vi "Add file.vi"(8 "error in (no error)":errorcluster, 9 "Insert in front":bool, 10 "File Path Control":path, 11 "MagLabGraph in":refnum<class "MagLabGraph.lvclass">) -> (0 "error out":errorcluster, 3 "MagLabGraph out":refnum<class "MagLabGraph.lvclass">)   [LabVIEW 2015, in "MagLabGraph.lvclass"]
uses:
  MagLabGraph.lvclass
  <vilib>/ActorFramework/Actor/Actor.lvclass/Actor.ctl
  <vilib>/ActorFramework/Message Enqueuer/Message Enqueuer.lvclass/Message Enqueuer.ctl
  MagLabGraph Messages/Add file Msg/Add file Msg.lvclass/Add file Msg.ctl
  MagLabGraph.lvclass/MagLabGraph.ctl
  <vilib>/ActorFramework/Message Enqueuer/Init from Existing Queue.vi
  <vilib>/ActorFramework/Time-Delayed Send Message/Time-Delayed Send Message.vi
  <vilib>/ActorFramework/Message Enqueuer/Message Enqueuer.lvclass
  MagLabGraph Messages/Add file Msg/Add file Msg.lvclass
  <vilib>/ActorFramework/Actor/Actor.lvclass
  Mag Lab Error Handler/Mag Lab Error Handler.lvclass
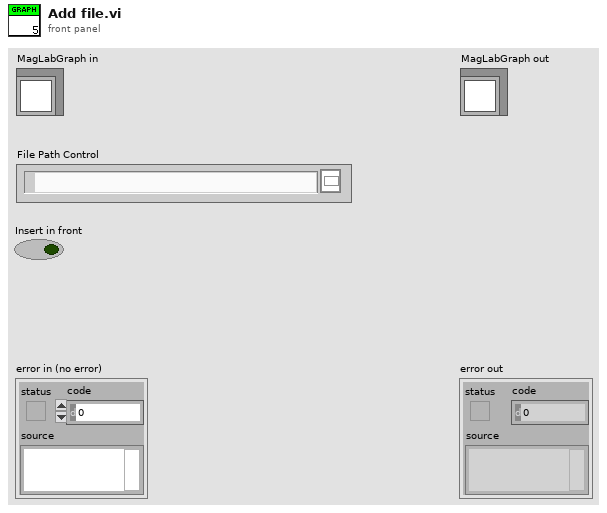
[diagram p1: front panel]
types:
  T1 = typedef "File_Group_Chan_Abbr.ctl" = cluster{"File Path Control":path, "Group":string, "Channel":string, "Abbreviated":string}
  T2 = cluster{"File Path Control":path, "Group":string, "Channel":string, "Abbreviated":string}[]
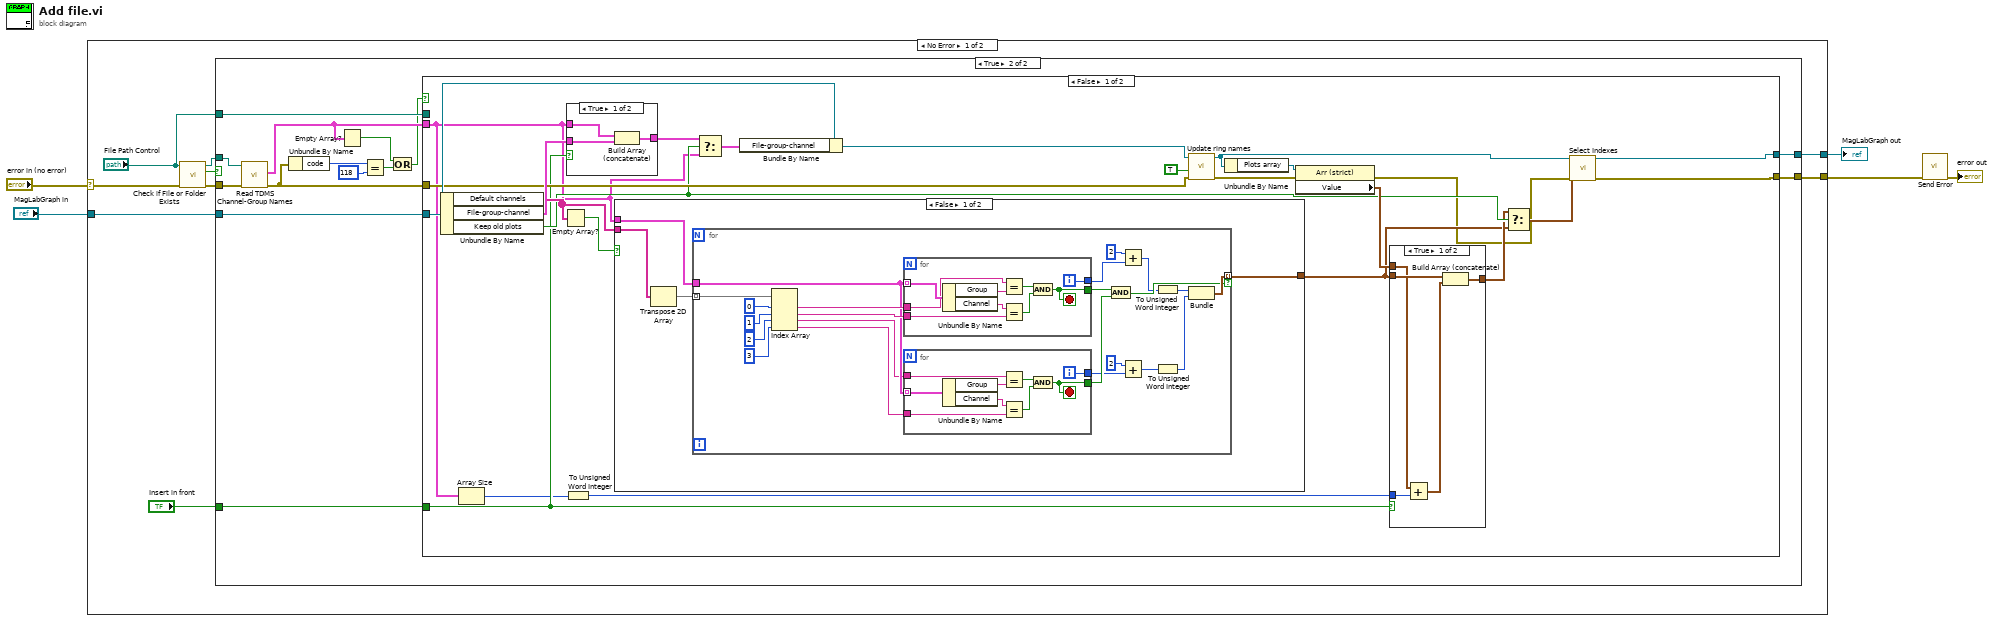
[diagram p0: block diagram]
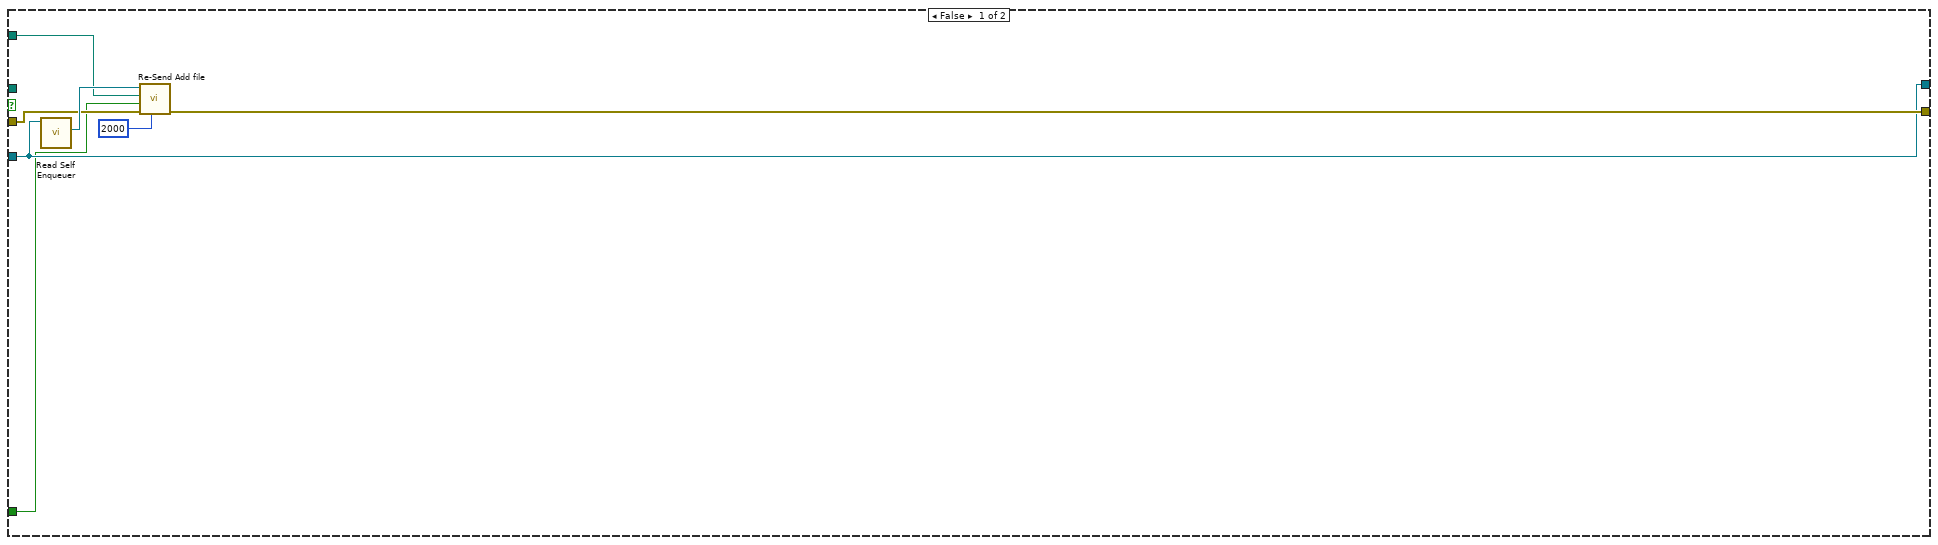
[diagram p2: hidden frame]
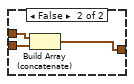
[diagram p3: hidden frame]
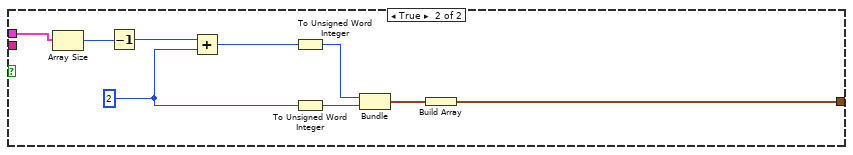
[diagram p4: hidden frame]
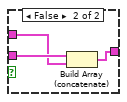
[diagram p5: hidden frame]
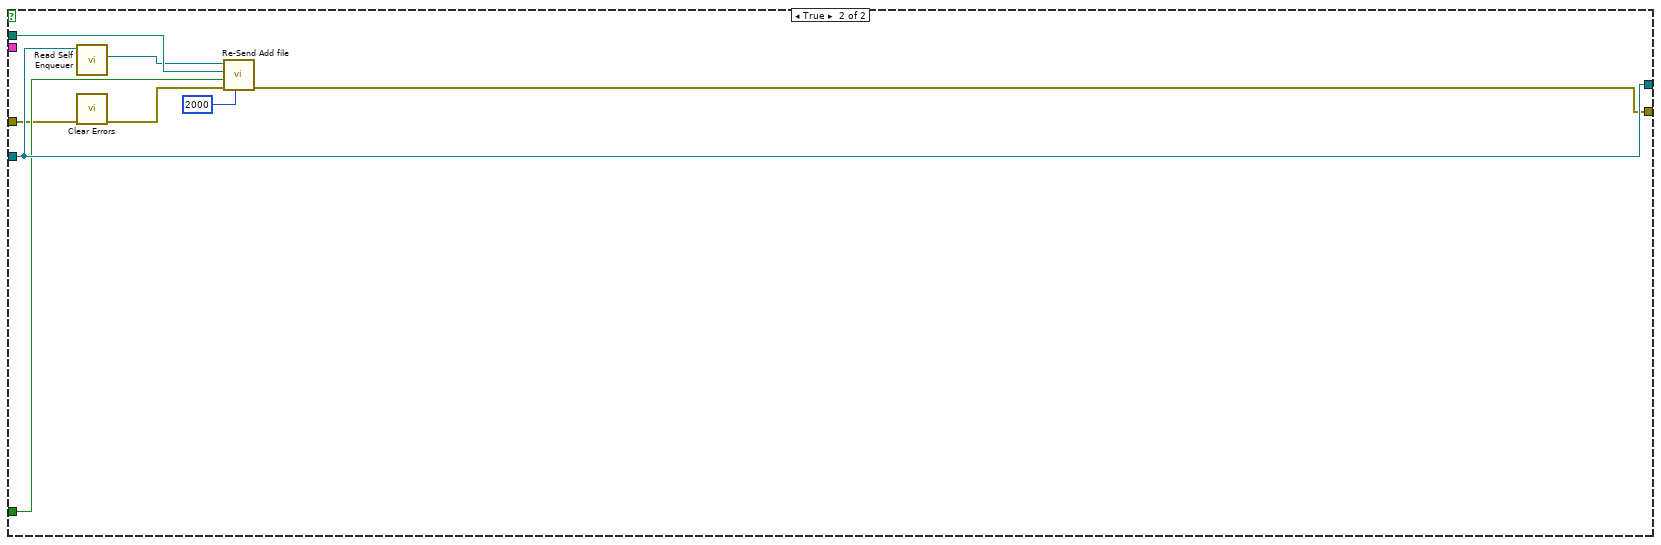
[diagram p6: hidden frame]
diagram:
  n1 = case shown="No Error" "error in (no error)" {
    selector: "error in (no error)" -> [w10 w136]
    tunnel: [w12 w136] -> w2
    tunnel: [w13 w135] -> w3
    tunnel: "MagLabGraph in" -> [w14 w135]
    frame No Error {
      n2 = call <vilib>:"Check if File or Folder Exists.vi"("error in (no error)"=w10, "path"="File Path Control") -> ("error out"=w9:errorcluster, "file or folder exists?"=w11:bool, "dup path"=w8:path)  [unwired: 7 in]
      n3 = case shown="True" w11 {
        tunnel: w9 -> [w20 w35]
        tunnel: w14 -> [w18 w34]
        tunnel: [w18 w33] -> w13
        tunnel: [w19 w32] -> w12
        tunnel: w8 -> [_ w31]
        tunnel: "File Path Control" -> [w17 w29]
        tunnel: "Insert in front" -> [w16 w30]
        frame False {
          n4 = call <vilib>:"Read Self Enqueuer.vi"("Actor"=w18) -> ("Self Enqueuer"=w21:refnum<class "Message Enqueuer.lvclass">)  [unwired: 10 in]
          n5 = call "Re-Send Add file.vi"("Milliseconds To Wait"=2000, "error in (no error)"=w20, "Insert in front"=w16, "File Path Control"=w17, "Message Enqueuer"=w21) -> ("error out"=w19:errorcluster)  [unwired: 5 in, 1 out]
        }
        frame True {
          n6 = call "Read TDMS Channel-Group Names.vi"("error in"=w35, "File Path Control"=w31) -> ("error out"=w23:errorcluster, "File-group-channel"=w28:T1[])  [unwired: 8 in]
          n7 = Unbundle By Name(w23) -> ("code"=w24:i32)
          n8 = Empty Array?(array=w28) -> (empty?=w27:bool)
          n9 = Equal?(x=w24, y=118) -> (x = y?=w22:bool)
          n10 = Or(x=w27, y=w22) -> (x .or. y?=w26:bool)
          n11 = case shown="False" w26 {
            tunnel: w34 -> [w59 w134]
            tunnel: [w39 w134] -> w33
            tunnel: w28 -> [w44 _]
            tunnel: [w37 w133] -> w32
            tunnel: w30 -> [w45 w132]
            tunnel: w29 -> [_ w131]
            tunnel: w23 -> [w52 w130]
            frame False {
              n12 = Unbundle By Name(w59) -> ("Default channels"=w50:string[][], "File-group-channel"=w55:T2, "Keep old plots"=w48:bool)
              n13 = Array Size(array=w44) -> (size(s)=w43:i32)
              n14 = Empty Array?(array=w50) -> (empty?=w51:bool)
              n15 = To Unsigned Word Integer(number=w43) -> (unsigned 16bit integer=w41:u16)
              n16 = case shown="True" w45 {
                tunnel: w55 -> [w121 w126]
                tunnel: w44 -> [w122 w125]
                tunnel: [w123 w124] -> w49
                frame True {
                  n17 = Build Array (concatenate)(w122, w121) -> (w123:T1[])
                }
                frame False {
                  n18 = Build Array (concatenate)(w126, w125) -> (w124:T1[])
                }
              }
              n19 = case shown="False" w51 {
                tunnel: w44 -> [w68 w113]
                tunnel: [w69 w114] -> w46
                tunnel: w50 -> [w71 _]
                frame False {
                  n20 = Transpose 2D Array(2D array=w71) -> (transposed array=w70:string[][])
                  n21 = for {
                    tunnel: w70 -> [w93] mode=indexing
                    tunnel: w68 -> [w86]
                    tunnel: [w79] -> w69 mode=indexing if=w78
                    n22 = Index Array(array=w93, index #1=0 ("index"), index #2=1 ("index"), index #3=2 ("index"), index #4=3 ("index")) -> (element #1=w88:string, element #2=w87:string, element #3=w85:string, element #4=w84:string)
                    n23 = for {
                      tunnel: w86 -> [w111] mode=indexing
                      tunnel: w88 -> [w109]
                      tunnel: w87 -> [w107]
                      tunnel: [w104] -> w83
                      tunnel: [w103] -> w76
                      i -> [w103]
                      stop <- w104 stop-if-true
                      n24 = Unbundle By Name(w111) -> ("Group"=w110:string, "Channel"=w108:string)
                      n25 = Equal?(x=w109, y=w110) -> (x = y?=w105:bool)
                      n26 = Equal?(x=w108, y=w107) -> (x = y?=w106:bool)
                      n27 = And(x=w105, y=w106) -> (x .and. y?=w104:bool)
                    }
                    n28 = for {
                      tunnel: w86 -> [w102] mode=indexing
                      tunnel: w85 -> [w100]
                      tunnel: w84 -> [w98]
                      tunnel: [w95] -> w82
                      tunnel: [w94] -> w73
                      i -> [w94]
                      stop <- w95 stop-if-true
                      n29 = Unbundle By Name(w102) -> ("Group"=w101:string, "Channel"=w99:string)
                      n30 = Equal?(x=w100, y=w101) -> (x = y?=w96:bool)
                      n31 = Equal?(x=w99, y=w98) -> (x = y?=w97:bool)
                      n32 = And(x=w96, y=w97) -> (x .and. y?=w95:bool)
                    }
                    n33 = And(x=w83, y=w82) -> (x .and. y?=w78:bool)
                    n34 = Add(x=2, y=w76) -> (x+y=w75:i32)
                    n35 = Add(x=2, y=w73) -> (x+y=w72:i32)
                    n36 = To Unsigned Word Integer(number=w75) -> (unsigned 16bit integer=w81:u16)
                    n37 = To Unsigned Word Integer(number=w72) -> (unsigned 16bit integer=w80:u16)
                    n38 = Bundle(w81, w80) -> (w79:cluster{u16, u16})  [unwired: 1 in]
                  }
                }
                frame True {
                  w112 = 2 ("x")
                  n39 = Array Size(array=w113) -> (size(s)=w118:i32)
                  n40 = Decrement(x=w118) -> (x-1=w116:i32)
                  n41 = Add(x=w116, y=w112) -> (x+y=w115:i32)
                  n42 = To Unsigned Word Integer(number=w115) -> (unsigned 16bit integer=w119:u16)
                  n43 = To Unsigned Word Integer(number=w112) -> (unsigned 16bit integer=w117:u16)
                  n44 = Bundle(w119, w117) -> (w120:cluster{u16, u16})  [unwired: 1 in]
                  n45 = Build Array(w120) -> (w114:cluster{u16, u16}[])
                }
              }
              n46 = Select(t=w49, s=w48, f=w44) -> (s? t:f=w42:T1[])
              n47 = Bundle By Name(cluster=w59, "File-group-channel"=w42) -> (w58:refnum<class "MagLabGraph.lvclass">)
              n48 = call "Update ring names.vi"("error in (no error)"=w52, "Update from File-group-channel"=TRUE, "MagLabGraph in"=w58) -> ("error out"=w56:errorcluster, "MagLabGraph out"=w40:refnum<class "MagLabGraph.lvclass">)  [unwired: 7 in]
              n49 = Unbundle By Name(w40) -> ("Plots array"=w57:refnum<vi>)
              n50 = property class="Arr (strict)"(reference=w57, error in=w56) -> (error out=w36:errorcluster, "Value"=w54:cluster{"X":u16, "Y":u16}[])  [unwired: 1 out]
              n51 = case shown="True" w45 {
                tunnel: w54 -> [w60 w66]
                tunnel: [w64 w67] -> w47
                tunnel: w46 -> [w63 w65]
                tunnel: w41 -> [w62 _]
                frame True {
                  n52 = Add(x=w60, y=w62) -> (x+y=w61:cluster{"X":u16, "Y":u16}[])
                  n53 = Build Array (concatenate)(w63, w61) -> (w64:cluster{"X":u16, "Y":u16}[])
                }
                frame False {
                  n54 = Build Array (concatenate)(w66, w65) -> (w67:cluster{"X":u16, "Y":u16}[])
                }
              }
              n55 = Select(t=w47, s=w48, f=w46) -> (s? t:f=w38:cluster{"X":u16, "Y":u16}[])
              n56 = call-dynamic "Select Indexes.vi"("error in (no error)"=w36, "Plot Indexes Array"=w38, "MagLabGraph in"=w40) -> ("error out"=w37:errorcluster, "MagLabGraph out"=w39:refnum<class "MagLabGraph.lvclass">)  [unwired: 7 in]
            }
            frame True {
              n57 = call <vilib>:"Read Self Enqueuer.vi"("Actor"=w134) -> ("Self Enqueuer"=w129:refnum<class "Message Enqueuer.lvclass">)  [unwired: 10 in]
              n58 = call <vilib>:"Clear Errors.vi"("error in (no error)"=w130) -> ("error out"=w127:errorcluster)  [unwired: 5 in, 1 out]
              n59 = call "Re-Send Add file.vi"("Milliseconds To Wait"=2000, "error in (no error)"=w127, "Insert in front"=w132, "File Path Control"=w131, "Message Enqueuer"=w129) -> ("error out"=w133:errorcluster)  [unwired: 5 in, 1 out]
            }
          }
        }
      }
    }
    frame Error {
    }
  }
  "MagLabGraph out" <- w3
  n60 = call "Send Error.vi"("error in (no error)"=w2) -> ("error out"=→"error out":errorcluster)  [unwired: 9 in, 1 out]
